vi "ScannerMirrorStatus.vi"() -> ()   [LabVIEW 2013]
panel:
  out "kinetics mirror":string
  out "kinetics scanner":string
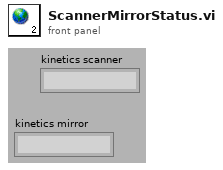
[diagram p1: front panel]
diagram:
